vi "Untitled 3.vi"() -> ()   [LabVIEW 2020]
uses:
  <userlib>/_NEVSTOP/Communicable State Machine(CSM)/_Support/Common/Trim Single line Text.vi
  <userlib>/_NEVSTOP/Communicable State Machine(CSM)/Communicable State Machine.lvlib
panel:
  in  "Tree":string(tree)
  out "Variant":variant
  out "size (in bytes)":i64
  out "XY Graph":T1(graph)
  out "offset (in bytes) (0)":i64
  in  "read line":bool
  in  "stop":bool
  out "data":string
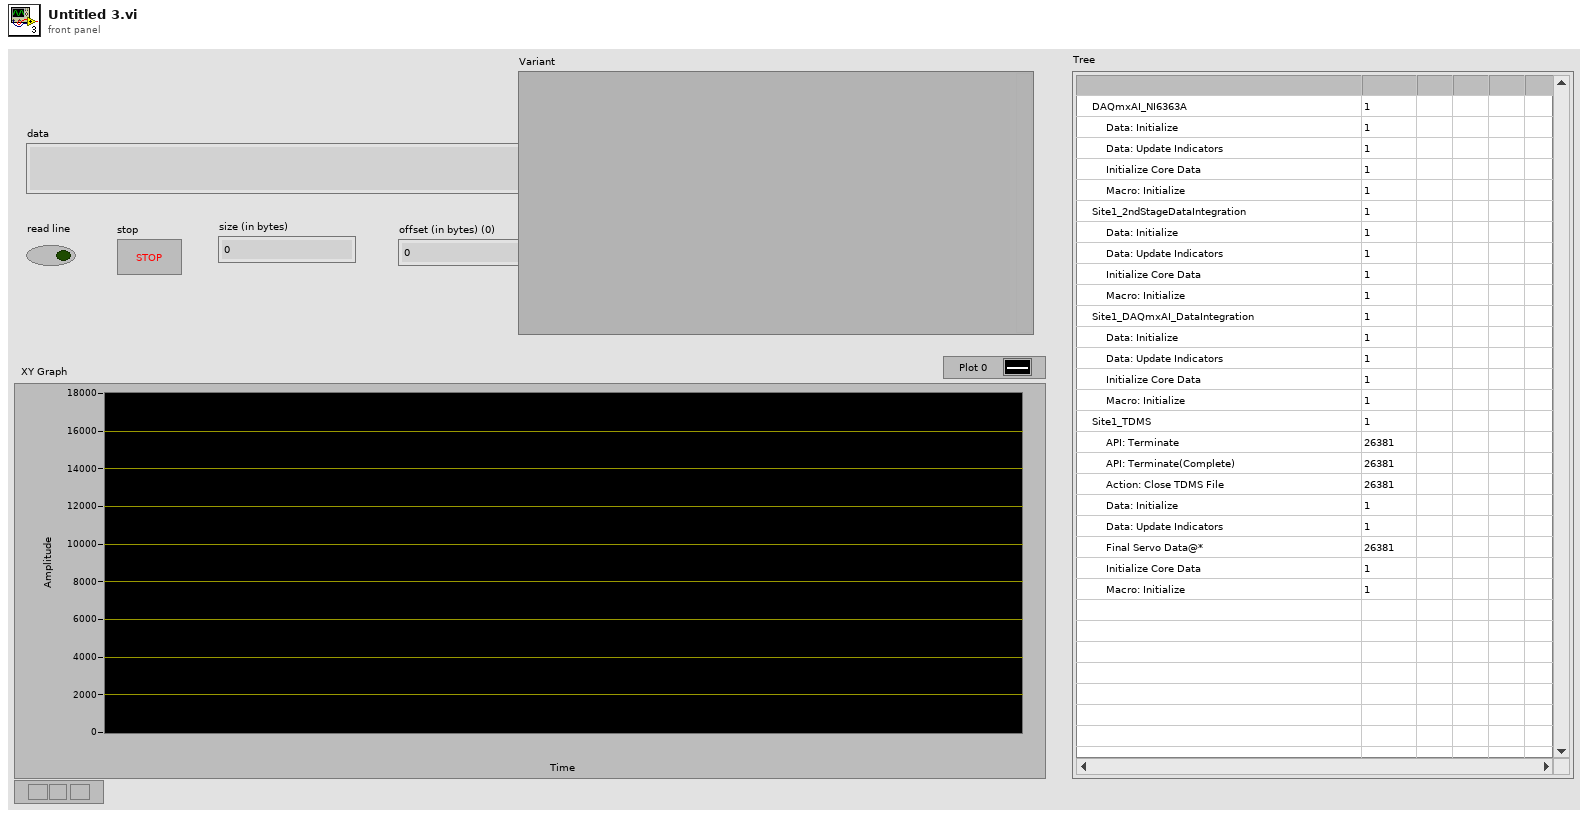
[diagram p1: front panel]
types:
  T1 = cluster{timestamp, "offset (in bytes) (0)":i64}[]
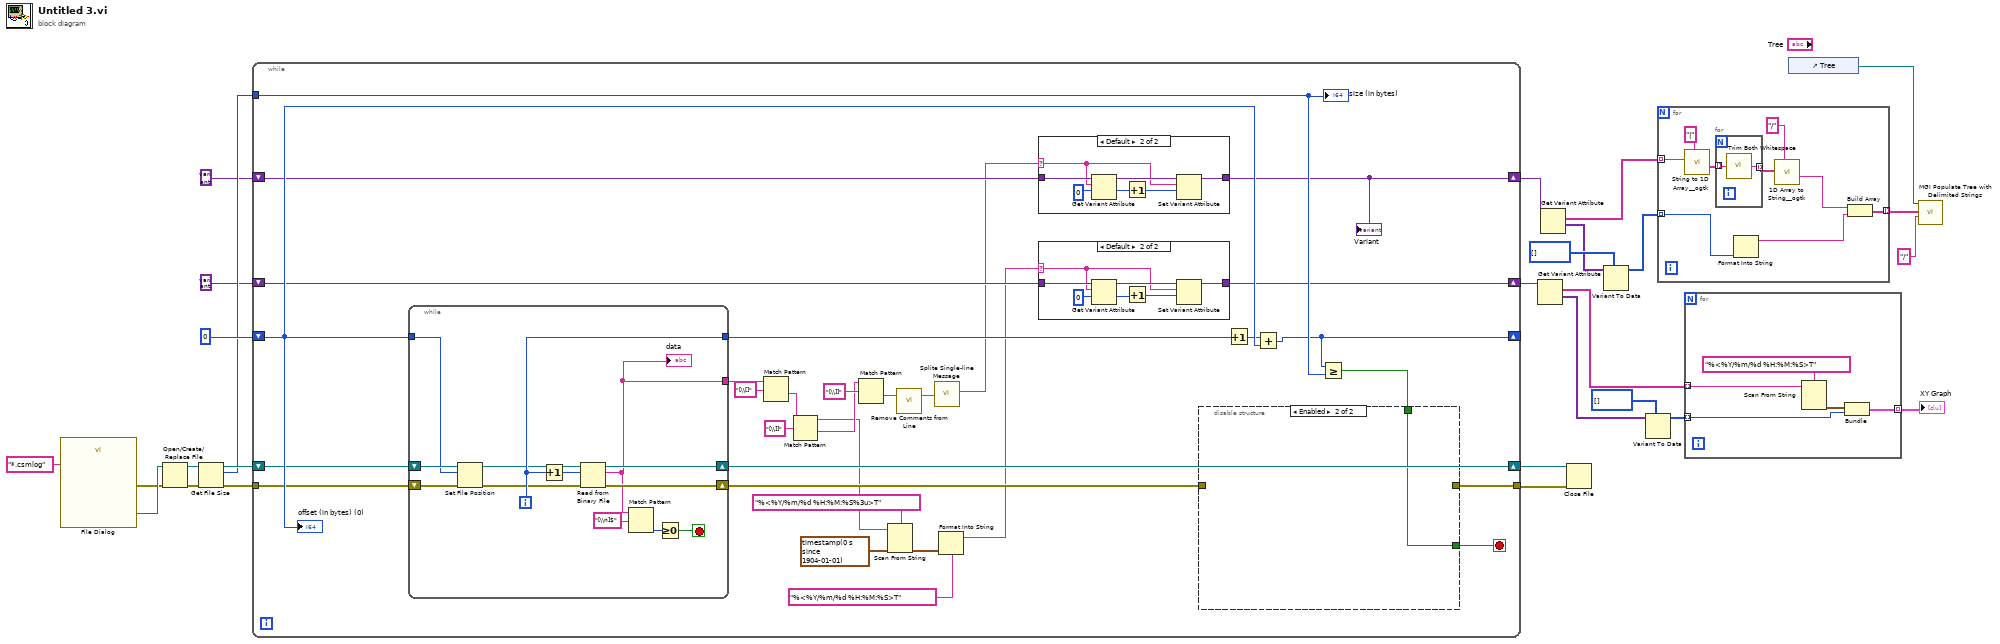
[diagram p0: block diagram]
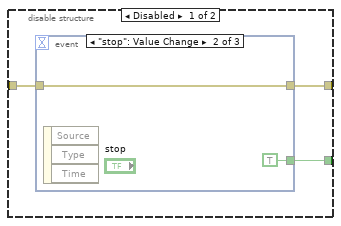
[diagram p4: hidden frame]
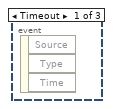
[diagram p5: hidden frame]
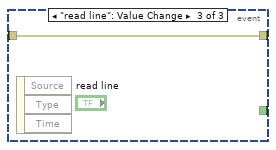
[diagram p6: hidden frame]
diagram:
  n1 = call "File Dialog"("pattern (all files)"="*.csmlog") -> ("selected path"=w3:path, "error out"=w2:errorcluster)  [unwired: 11 in, 2 out]
  n2 = Open/Create/Replace File(file path (use dialog)=w3, error in=w2) -> (refnum out=w27:refnum<file>, error out=w26:errorcluster)  [unwired: 4 in, 1 out]
  n3 = Get File Size(file=w27, error in=w26) -> (refnum out=w24:refnum<file>, size (in bytes)=w20:i64, 0:w23:errorcluster)
  n4 = while {
    shift-right: [w58] -> w21
    shift-left: w24 -> [w52]
    tunnel: [w55] -> w22
    shift-right: [w41] -> _
    shift-left: i64 0 ("offset (in bytes) (0)") -> [w53]
    tunnel: w23 -> [w51]
    tunnel: w20 -> [w49]
    shift-right: [w42] -> w13
    shift-left: variant -> [w43]
    shift-right: [w35] -> w9
    shift-left: variant -> [w36]
    stop <- w56 stop-if-true
    n5 = while {
      shift-right: [w86] -> w54
      shift-left: w51 -> [w80]
      shift-right: [w87] -> w58
      shift-left: w52 -> [w77]
      tunnel: [w81] -> w57
      tunnel: w53 -> [w76]
      tunnel: [w75] -> w47
      i -> [w81]
      stop <- w83 stop-if-true
      n6 = Set File Position(offset (in bytes) (0)=w76, refnum=w77, error in=w80) -> (refnum out=w78:refnum<file>, error out=w79:errorcluster)  [unwired: 1 in]
      n7 = Increment(x=w81) -> (x+1=w82:i32)
      n8 = Read from Binary File(8:w79, 10:w82, 11:w78) -> (0:w86:errorcluster, 2:w75:string, 3:w87:refnum<file>)  [unwired: 3 in, 1 out]
      "data" <- w75
      n9 = Match Pattern(string=w75, regular expression="[\\n]$") -> (offset past match=w84:i32)  [unwired: 1 in, 3 out]
      n10 = Greater Or Equal To 0?(x=w84) -> (x >= 0?=w83:bool)
    }
    n11 = Match Pattern(string=w47, regular expression="[\\[]") -> (after substring=w45:string)  [unwired: 1 in, 3 out]
    n12 = Match Pattern(string=w45, regular expression="[\\]]") -> (before substring=w33:string, after substring=w38:string)  [unwired: 1 in, 2 out]
    n13 = Match Pattern(string=w38, regular expression="[\\]]") -> (after substring=w37:string)  [unwired: 1 in, 3 out]
    n14 = Scan From String(format string="%<%Y/%m/%d %H:%M:%S%3u>T", input string=w33, default 1=timestamp(0 s since 1904-01-01)) -> (output 1=w30:timestamp)  [unwired: 2 in, 3 out]
    n15 = call <userlib>:"Remove Comments from Line.vi"("single-line text"=w37) -> ("single-line text without comments"=w40:string)  [unwired: 2 in]
    n16 = call <userlib>:"Splite Single-line Message.vi"("single-line text"=w40) -> ("state"=w34:string)  [unwired: 6 in, 3 out]
    n17 = Format Into String(format string="%<%Y/%m/%d %H:%M:%S>T", w30) -> (resulting string=w28:string)  [unwired: 2 in, 1 out]
    n18 = case shown="Default" w34 {
      selector: w34 -> [_ w60]
      tunnel: w36 -> [w59 w66]
      tunnel: [w59 w62] -> w35
      frame "" {
      }
      frame Default {
        n19 = Get Variant Attribute(Variant=w66, name=w60, default value (empty Variant)=i64 0 ("offset (in bytes) (0)")) -> (duplicate Variant=w63:variant, value=w64:i64)  [unwired: 1 in, 2 out]
        n20 = Increment(x=w64) -> (x+1=w61:i64)
        n21 = Set Variant Attribute(Variant=w63, name=w60, value=w61) -> (Variant out=w62:variant)  [unwired: 1 in, 2 out]
      }
    }
    "Variant" <- w35
    n22 = case shown="Default" w28 {
      selector: w28 -> [_ w68]
      tunnel: w43 -> [w67 w74]
      tunnel: [w67 w70] -> w42
      frame "" {
      }
      frame Default {
        n23 = Get Variant Attribute(Variant=w74, name=w68, default value (empty Variant)=i64 0 ("offset (in bytes) (0)")) -> (duplicate Variant=w71:variant, value=w72:i64)  [unwired: 1 in, 2 out]
        n24 = Increment(x=w72) -> (x+1=w69:i64)
        n25 = Set Variant Attribute(Variant=w71, name=w68, value=w69) -> (Variant out=w70:variant)  [unwired: 1 in, 2 out]
      }
    }
    n26 = Increment(x=w57) -> (x+1=w50:i32)
    n27 = Add(x=w50, y=w53) -> (x+y=w41:i64)
    n28 = Greater Or Equal?(x=w41, y=w49) -> (x >= y?=w48:bool)
    n29 = disable-structure shown="Enabled" {
      disable-tunnel: [w90 w94] -> w56
      disable-tunnel: [w89 _] -> w55
      disable-tunnel: w54 -> [w88 _]
      disable-tunnel: w48 -> [_ w94]
      frame Disabled {
        n30 = event shown="[1] \"stop\": Value Change" {
          selector: _ -> [_ _ _]
          dyn-events: _ -> [_ _ _]
          timeout: _ -> [_ _ _]
          tunnel: [_ TRUE ("stop") _] -> w90
          tunnel: [_ w92 w93] -> w89
          tunnel: w88 -> [_ w92 w93]
          event Timeout {
            n31 = event-data() -> ()  [unwired: 1 in, 3 out]
          }
          event "stop": Value Change {
            n32 = event-data() -> ()  [unwired: 1 in, 3 out]
          }
          event "read line": Value Change {
            n33 = event-data() -> ()  [unwired: 1 in, 3 out]
          }
        }
      }
      frame Enabled {
      }
    }
    "offset (in bytes) (0)" <- w53
    "size (in bytes)" <- w49
  }
  n34 = Get Variant Attribute(Variant=w13) -> (names=w15:string[], values=w16:variant[])  [unwired: 3 in, 2 out]
  n35 = Get Variant Attribute(Variant=w9) -> (names=w8:string[], values=w10:variant[])  [unwired: 3 in, 2 out]
  n36 = Close File(refnum=w21, error in=w22) -> ()  [unwired: 2 out]
  n37 = Variant To Data(type=i64[] [] ("offset (in bytes) (0)"), Variant=w10) -> (data=w7:i64[])  [unwired: 1 in, 1 out]
  n38 = Variant To Data(type=i64[] [] ("offset (in bytes) (0)"), Variant=w16) -> (data=w17:i64[])  [unwired: 1 in, 1 out]
  n39 = for {
    tunnel: w8 -> [w103] mode=indexing
    tunnel: w7 -> [w97] mode=indexing
    tunnel: [w95] -> w6 mode=indexing
    n40 = call <userlib>:"String to 1D Array__ogtk.vi"("delimiter (Tab)"="|", "string"=w103) -> ("Array of Strings"=w101:string[])  [unwired: 9 in]
    n41 = for {
      tunnel: w101 -> [w105] mode=indexing
      tunnel: [w104] -> w100 mode=indexing
      n42 = call <userlib>:"Trim Both Whitespace.vi"("string"=w105) -> ("trimmed string"=w104:string)  [unwired: 1 in]
    }
    n43 = Format Into String(w97) -> (resulting string=w96:string)  [unwired: 3 in, 1 out]
    n44 = call <userlib>:"1D Array to String__ogtk.vi"("delimiter (Tab)"="/", "Array of Strings"=w100) -> ("delimited string"=w98:string)  [unwired: 9 in]
    n45 = Build Array(w98, w96) -> (w95:string[])
  }
  n46 = for {
    tunnel: w15 -> [w109] mode=indexing
    tunnel: w17 -> [w107] mode=indexing
    tunnel: [w106] -> w18 mode=indexing
    n47 = Scan From String(format string="%<%Y/%m/%d %H:%M:%S>T", input string=w109) -> (output 1=w108:timestamp)  [unwired: 3 in, 3 out]
    n48 = Bundle(w108, "offset (in bytes) (0)"=w107) -> (w106:cluster{timestamp, "offset (in bytes) (0)":i64})  [unwired: 1 in]
  }
  "XY Graph" <- w18
  n49 = control-ref of="Tree"() -> (w4:refnum<vi>)
  n50 = call <userlib>:"MGI Populate Tree with Delimited Strings.vi"("Delimiter"="/" ("delimiter (Tab)"), "Items (Delimited)"=w6, "Tree Control"=w4) -> ()  [unwired: 6 in, 3 out]
